vi "DB Tools Build Insert Query.vi"(4 "num parameters":i32, 5 "error in (no error)":errorcluster, 6 "columns":string[](array[string]), 7 "table name":string) -> (0 "error out":errorcluster, 2 "insert query":string)   [LabVIEW 2013, in "NI_Database_API_64.lvlib"]
doc: "Builds the SQL INSERT statement using the specified table name, columns array, and num parameters."
uses:
  NI_Database_API_64.lvlib
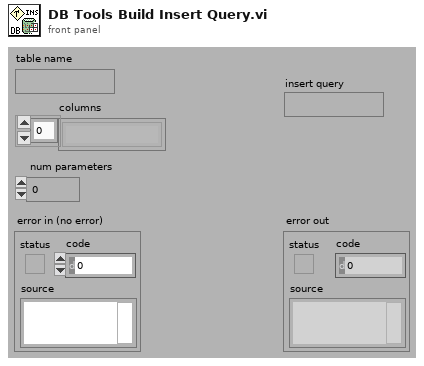
[diagram p1: front panel]
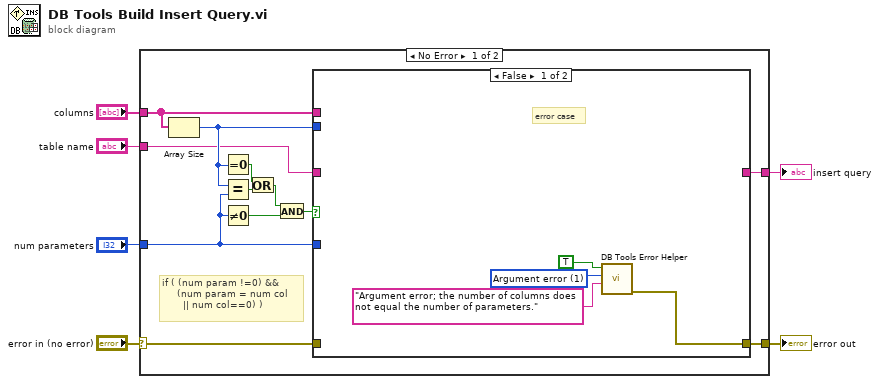
[diagram p0: block diagram]
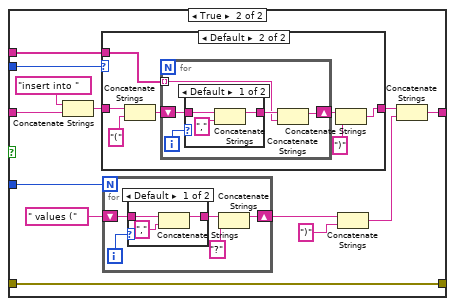
[diagram p2: hidden frame]
diagram:
  n1 = case shown="No Error" "error in (no error)" {
    selector: "error in (no error)" -> [w12 w62]
    tunnel: [w11 w62] -> w5
    tunnel: "columns" -> [w10 _]
    tunnel: "num parameters" -> [w9 _]
    tunnel: [w8 _] -> w2
    tunnel: "table name" -> [w7 _]
    frame No Error {
      # "if ( (num param !=0) &&\n     (num param = num col \n       || num col==0) )"
      n2 = Array Size(array=w10) -> (size(s)=w13:i32)
      n3 = Equal To 0?(x=w13) -> (x = 0?=w18:bool)
      n4 = Equal?(x=w13, y=w9) -> (x = y?=w14:bool)
      n5 = Not Equal To 0?(x=w9) -> (x != 0?=w17:bool)
      n6 = Or(x=w18, y=w14) -> (x .or. y?=w16:bool)
      n7 = And(x=w16, y=w17) -> (x .and. y?=w15:bool)
      n8 = case shown="False" w15 {
        tunnel: w10 -> [_ w32]
        tunnel: w13 -> [_ w31]
        tunnel: w9 -> [_ w29]
        tunnel: w12 -> [_ w25]
        tunnel: [w22 w25] -> w11
        tunnel: [_ w24] -> w8
        tunnel: w7 -> [_ w23]
        frame False {
          w20 = 1 items=["No error", "Argument error", "Memory is full", "Out of zone", "End of file", "File already open", "Generic file I/O error", "File not found", "File permission error", "Disk is full", "Duplicate path", "Too many files open", "System feature not enabled", "Resource file not found", "Cannot add resource", "Resource not found", "Image not found", "Image memory error", "Pen does not exist", "Config type invalid", "Config token not found", "Config parse error", "Config memory error", "Bad external code format", "Bad external code offset", "External code not present", "Null window", "Destroy window error", "Null menu", "Print aborted", "Bad print record", "Print driver error", "Windows error during printing", "Memory error during printing", "Print dialog error", "Generic print error", "Invalid device refnum", "Device not found", "Device parameter error", "Device unit error", "Cannot open device", "Device call aborted", "Generic error", "Cancelled by user", "Object ID too low", "Object ID too high", "Object not in heap", "Unknown heap", "Unknown object (invalid DefProc)", "Unknown object (DefProc not in table)", "Message out of range", "Invalid (null) method", "Unknown message", "Manager call not supported", "Bad address", "Network operation in progress", "Network operation timed out", "Connection is busy", "Network attribute not supported", "Network error", "Address in use", "System out of memory", "Connection aborted", "Connection refused", "Not connected", "Already connected", "Connection closed", "Initialization error (interapplication manager)", "Bad occurrence", "Wait on unbound occurrence handler", "Occurrence queue overflow", "Datalog type conflict", "Unused", "Unrecognized type (interapplication manager)", "Memory corrupt", "Failed to make temporary DLL", "Old CIN version", "Drag socket not found", "Failed to load drop-object", "Failed to register OLE object", "Failed to release OLE object", "Format specifier type mismatch", "Unknown format specifier", "Too few format specifiers", "Too many format specifiers", "Scan failed", "Newer CIN version", "Error converting to variant", "Runtime menu error", "Password tampered", "Variant attribute not found", "Incompatible variant data type", "Event data is not available", "Event Store is not present", "Occurrence is not found", "Event Queue is not created", "Event info is not available", "Refnum passed is NULL", "Error retrieving Class GUID", "Error retrieving CoClass GUID", "Error retrieving TypeLib GUID.", "Bad built application magic bytes.", "Specific driver is different from the specific driver associated with the Logical Name.", "There is no session opened to the class driver.", "Max Error", "MAX - Error with config objects", "MAX - Error loading configuration", "MAX - Group not supported"]
          # "error case"
          n9 = call "DB Tools Error Helper.vi"("source"="Argument error; the number of columns does not equal the number of parameters.", "code"=w20, "status"=TRUE) -> ("error out"=w22:errorcluster)  [unwired: 1 in, 7 out]
        }
        frame True {
          n10 = Concatenate Strings("insert into " ("Substring"), w23) -> (w34:string)
          n11 = case shown="Default" w31 {
            tunnel: w32 -> [_ w52]
            tunnel: [w45 w46] -> w35
            tunnel: w34 -> [w45 w51]
            frame 0 {
              # "if the columns\narray is empty"
            }
            frame Default {
              n12 = Concatenate Strings(w51, "(" ("Substring")) -> (w49:string)
              n13 = for {
                tunnel: w52 -> [w54] mode=indexing
                shift-right: [w53] -> w48
                shift-left: w49 -> [w56]
                i -> [w57]
                n14 = case shown="Default" w57 {
                  tunnel: w56 -> [w60 w61]
                  tunnel: [w58 w61] -> w55
                  frame Default {
                    n15 = Concatenate Strings(w60, "," ("Substring")) -> (w58:string)
                  }
                  frame 0 {
                  }
                }
                n16 = Concatenate Strings(w55, w54) -> (w53:string)
              }
              n17 = Concatenate Strings(w48, ")" ("Substring")) -> (w46:string)
            }
          }
          n18 = for {
            N: w29 -> [_]
            shift-right: [w37] -> w27
            shift-left: " values (" ("Substring") -> [w39]
            i -> [w40]
            n19 = case shown="Default" w40 {
              tunnel: w39 -> [w43 w44]
              tunnel: [w41 w44] -> w38
              frame Default {
                n20 = Concatenate Strings(w43, "," ("Substring")) -> (w41:string)
              }
              frame 0 {
              }
            }
            n21 = Concatenate Strings(w38, "?") -> (w37:string)
          }
          n22 = Concatenate Strings(w27, ")" ("Substring")) -> (w26:string)
          n23 = Concatenate Strings(w35, w26) -> (w24:string)
        }
      }
    }
    frame Error {
    }
  }
  "error out" <- w5
  "insert query" <- w2
